vi "Process.vi"(8 "error in (no error)":errorcluster, 10 "pound in":refnum<class "Pound.lvclass">, 11 "qbus in":refnum<class "Qbus.lvclass">) -> (0 "error out":errorcluster)   [LabVIEW 2017, in "CmsAcquisition.lvlib"]
doc: "This process acquires waveforms from channels on NI 9230 and NI 9232 C Series modules. This process transfers data from a device-specific FPGA bitfile that reads samples directly from the FPGA at the sampling rate configured for the device."
uses:
  <vilib>/addons/InsightCM/Devices/Shared/Cms/CmsAcquisition/CmsAcquisition.lvlib
  <vilib>/addons/Qbus/Qbus.lvclass
  <vilib>/NI/Software Watchdog/Pound/Pound.lvclass
  <vilib>/addons/InsightCM/Devices/Shared/Cms/CmsAcquisition/controls/Configuration.ctl
  <vilib>/addons/InsightCM/Devices/Shared/Cms/CmsAcquisition/controls/TachometerConfig.ctl
  <vilib>/addons/InsightCM/Devices/Shared/Cms/CmsAcquisition/controls/FixedSizeArrays.ctl
  <vilib>/LabVIEW Targets/FPGA/cRIO/shared/nicrio_ModuleControls/nicrio_cRIO-9232_ConfigModeRing.ctl
  <vilib>/addons/InsightCM/Devices/Shared/Cms/cRIOWfmAcq/subVIs/RIO Wfm Cust Ctrls/rwfm_SamplingInfo.ctl
  <vilib>/addons/InsightCM/Devices/Shared/Cms/CmsAcquisition/controls/Group.ctl
  <vilib>/addons/InsightCM/Devices/Shared/Cms/CmsAcquisition/controls/Channel.ctl
  <vilib>/addons/InsightCM/Utilities/Analysis/Vibration/controls/HighPassFilterState.ctl
  <vilib>/addons/InsightCM/Devices/Shared/Cms/CmsAcquisition/controls/BurstMode.ctl
  <vilib>/addons/InsightCM/Devices/Shared/Cms/CmsAcquisition/controls/State.ctl
  <vilib>/addons/InsightCM/Devices/Shared/Common/DataFlow/controls/Type.ctl
  <vilib>/addons/InsightCM/Devices/Shared/Cms/CmsAcquisition/controls/StopAcquisitionResponse.ctl
  <vilib>/addons/InsightCM/Devices/Shared/Cms/cRIOWfmAcq/cRIOWfmLib.lvlib
  <vilib>/addons/TraceLogger/TraceLogger.lvlib
  <vilib>/NI/Software Watchdog/Watchdog/Watchdog.lvclass
  <vilib>/addons/InsightCM/Devices/Shared/Common/FpgaBitfileManager/FpgaBitfileManager.lvlib
  <vilib>/addons/InsightCM/Devices/Shared/Common/DataFlow/DataFlow.lvlib
  <vilib>/addons/InsightCM/Utilities/GlobalConfiguration/GlobalConfiguration.lvlib
  <vilib>/addons/InsightCM/Devices/Shared/Common/DataEventCreator/DataEventCreator.lvlib
  <vilib>/addons/InsightCM/Devices/Shared/Common/ServerComm/ServerComm.lvlib
  <vilib>/addons/InsightCM/Utilities/Analysis/Vibration/VibrationAnalysisFunctions.lvlib
  <vilib>/addons/InsightCM/Devices/Shared/Cms/CmsBurstMode/BurstMode.lvlib
  <vilib>/addons/InsightCM/Devices/Shared/Cms/CmsDataEventCreator/CmsDataEventCreator.lvlib
  <vilib>/addons/InsightCM/Devices/Shared/Cms/DAQmx/TSNcDAQ_AI.lvlib
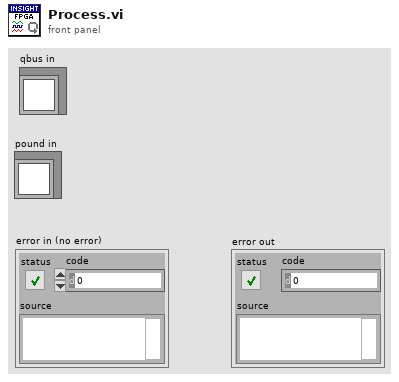
[diagram p1: front panel]
types:
  T1 = typedef "CmsAcquisition.lvlib/State.ctl" = enum16{"Unconfigured", "Configured", "Acquiring", "Stopped", "BurstMode"}
  T2 = typedef "CmsAcquisition.lvlib/Configuration.ctl" = cluster{"Acq":bool, "NumberOfModules":i16, "Dynamic FPGA VI Ref":refnum<k20>, "KeyphasorX3":T3[], "FixedSizeX32":T4, "SamplingInfo":T6, "Normal Mode Sample Rate":dbl, "BlockSize (sec)":dbl, "Samples To Read (per chan)":i32, "RunningAcquisitionLength":dbl, "Settling Time":dbl, "Fpga Tach Buffer Size (samples)":i32, "Waveform Groups":T7[], "Acquisition Block Number":i32, "Device Name":string, "ValidConfig":bool, "Last Dynamic Module":string, "HighPassFilterState":T9[], "Low Frequency Cutoff":dbl[], "BurstMode":T10, "DAQ task":refnum<k21>}
  T3 = typedef "CmsAcquisition.lvlib/TachometerConfig.ctl" = cluster{"slope":enum16{"falling", "rising"}, "threshold":dbl, "hysteresis":dbl}
  T4 = typedef "CmsAcquisition.lvlib/FixedSizeArrays.ctl" = cluster{"EnabledChannels":bool[], "Sensitivity":dbl[], "InputConfig":T5[]}
  T5 = typedef "nicrio_cRIO-9232_ConfigModeRing.ctl" = u8
  T6 = typedef "cRIOWfmLib.lvlib/rwfm_SamplingInfo.ctl" = cluster{"Number of Channels":i32, "Sampling Rate":dbl, "Channels":string[], "Units":string[], "Offsets":sgl[]}
  T7 = typedef "CmsAcquisition.lvlib/Group.ctl" = cluster{"Name":string, "Speed Reference":string, "Channels":T8[]}
  T8 = typedef "CmsAcquisition.lvlib/Channel.ctl" = cluster{"Name":string}
  T9 = typedef "VibrationAnalysisFunctions.lvlib/HighPassFilterState.ctl" = cluster{"designed":bool, "IIR Filter Cluster":cluster{"filter structure":enum32{"IIR 2nd Order", "IIR 4th Order"}, "Reverse Coefficients":dbl[], "Forward Coefficients":dbl[]}, "Filter State":dbl[]}
  T10 = typedef "CmsAcquisition.lvlib/BurstMode.ctl" = cluster{"Acquisition Time":dbl, "Sample Rate":dbl, "Collection Reason":string}
  T11 = typedef "DataFlow.lvlib/Type.ctl" = enum16{"High Rate", "Low Rate", "Burst Mode"}
  T12 = typedef "CmsAcquisition.lvlib/StopAcquisitionResponse.ctl" = cluster{"Reason":string, "Acquisition Stopped":bool, "State":variant}
  T13 = typedef "DataEventCreator.lvlib/RegisterDataSets.ctl" = cluster{"DataGroup":string, "DataSets":T14[]}
  T14 = typedef "CmsDataEventCreator.lvlib/DataSetRegistry.ctl" = cluster{"ChannelName":string, "DataSetType":T15, "DoNotWriteToDB":bool, "ParentName":string, "CalculateOnServer":bool}
  T15 = typedef "DataEvent.lvlib/DataSetType.ctl" = enum16{"Waveform", "SpeedProfile", "ThermalImage", "EmsaSweep"}
  T16 = typedef "DataFlow.lvlib/Data.ctl" = cluster{"DataGroup":string, "Waveforms":T17, "Map":T18, "Type":T11}
  T17 = typedef "wfmSGL_DVR.ctl" = refnum<data-value>
  T18 = typedef "PointValueMap.lvlib/PointMap.ctl" = refnum<data-value>
  T19 = typedef "CmsAcquisition.lvlib/StopAcquisitionRequest.ctl" = cluster{"Reason":string, "State":variant}
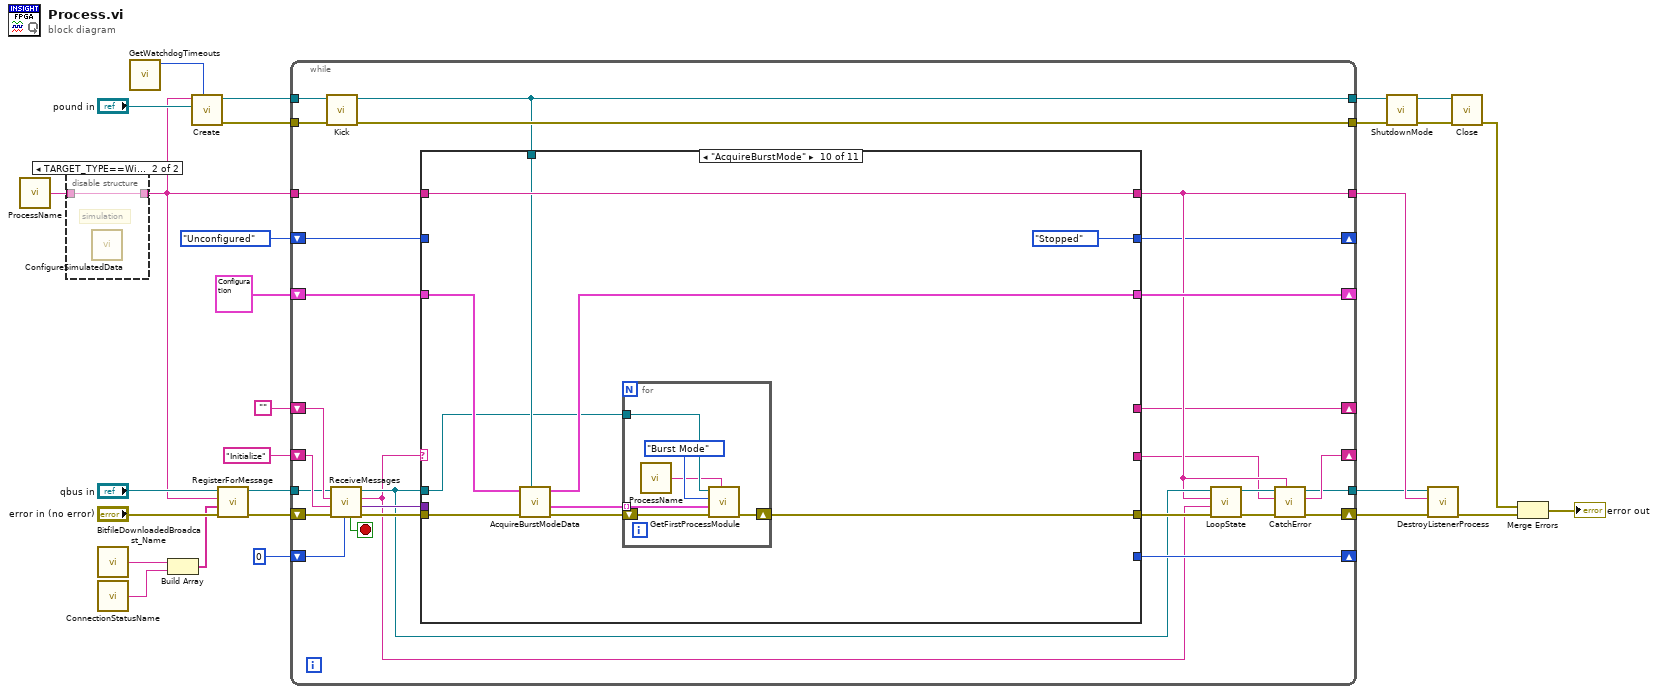
[diagram p0: block diagram]
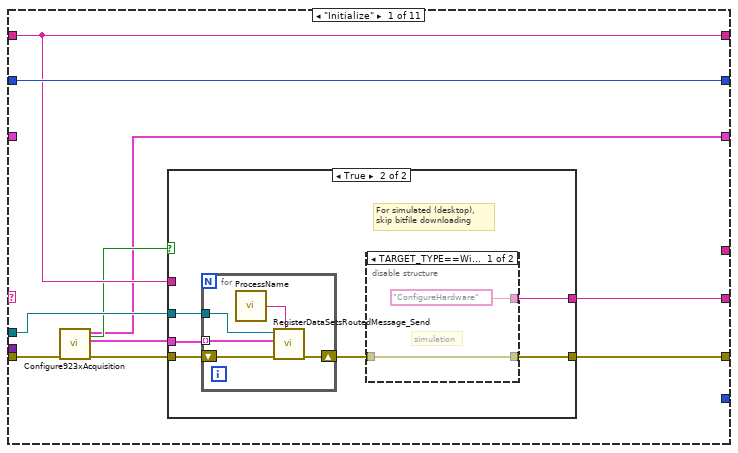
[diagram p3: hidden frame]
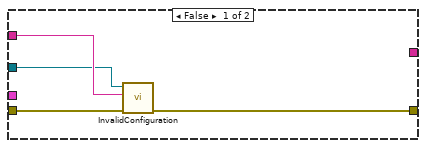
[diagram p4: hidden frame]
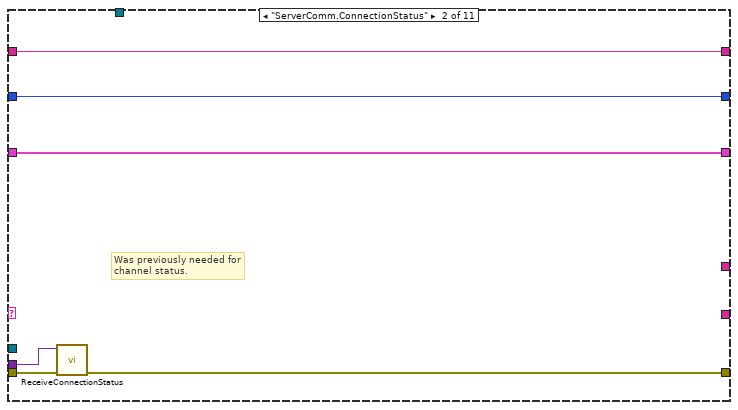
[diagram p6: hidden frame]
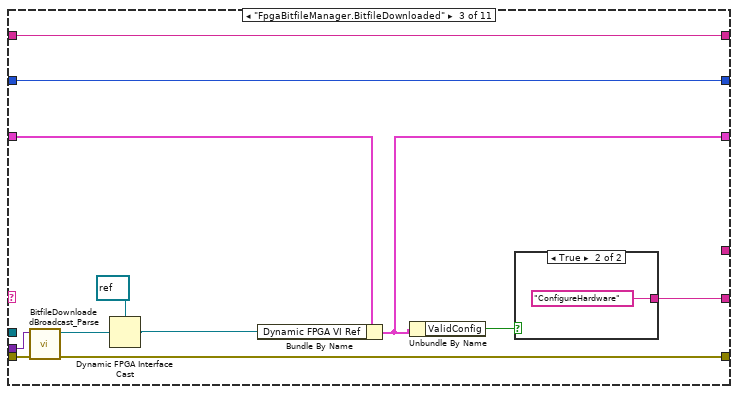
[diagram p7: hidden frame]
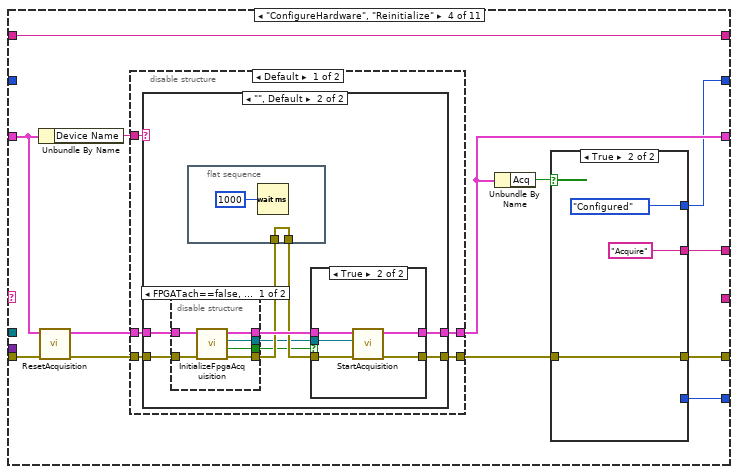
[diagram p9: hidden frame]
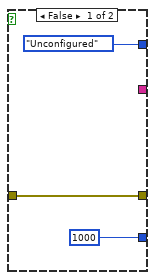
[diagram p10: hidden frame]
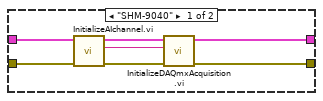
[diagram p11: hidden frame]
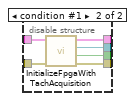
[diagram p13: hidden frame]
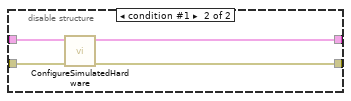
[diagram p14: hidden frame]
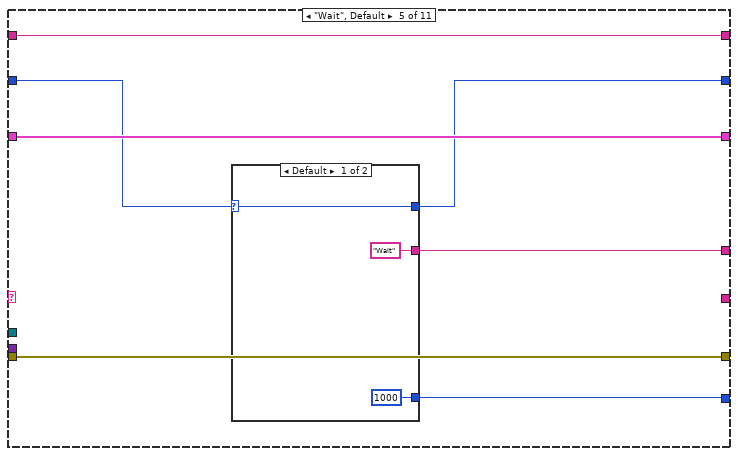
[diagram p15: hidden frame]
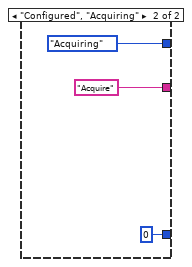
[diagram p16: hidden frame]
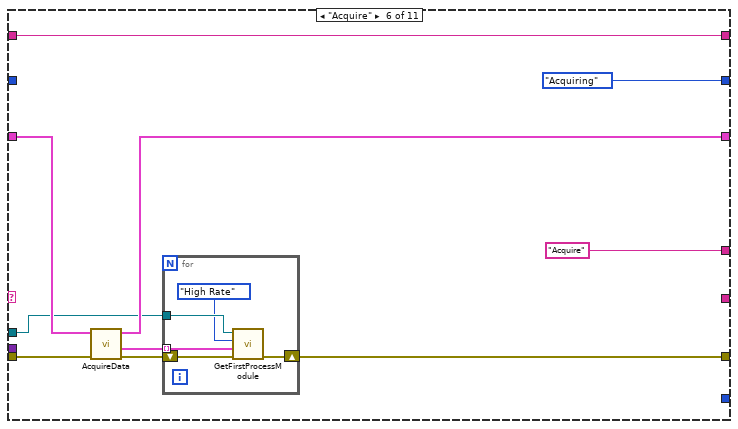
[diagram p17: hidden frame]
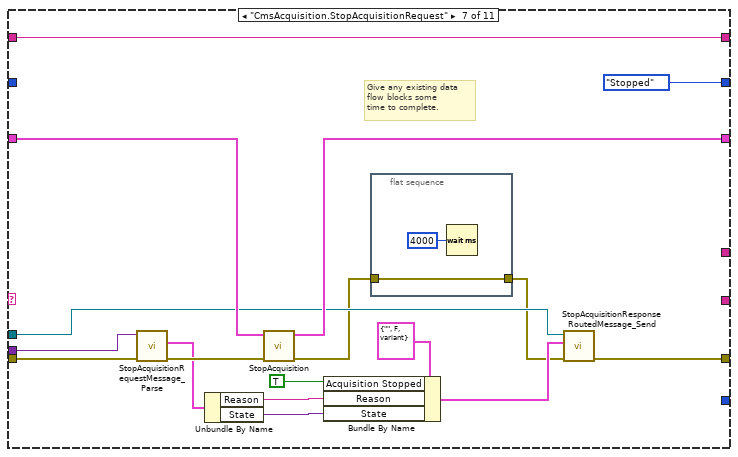
[diagram p18: hidden frame]
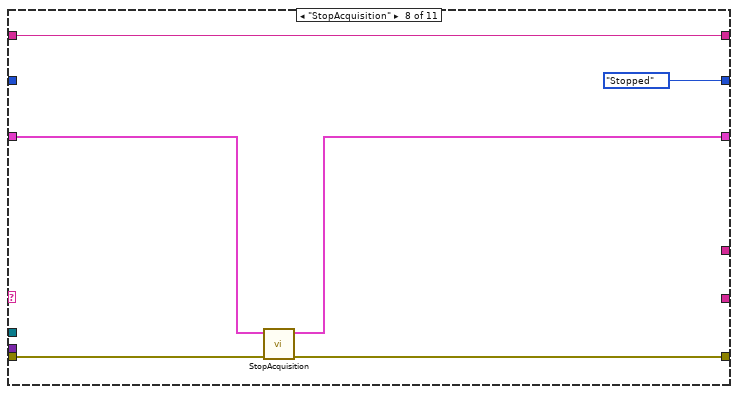
[diagram p19: hidden frame]
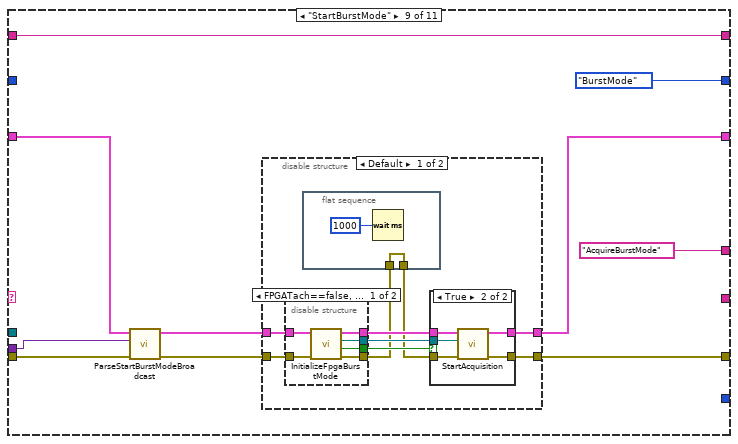
[diagram p20: hidden frame]
diagram:
  n1 = call <vilib>:"ProcessName.vi"() -> ("process name"=w6:string)  [unwired: 5 in]
  n2 = disable-structure shown="TARGET_TYPE==Windows" {
    disable-tunnel: [w29 w30] -> w7
    disable-tunnel: w6 -> [w29 w30]
    frame condition #0 (active) {
    }
    frame condition #1 {
      # "simulation"
      n3 = call <vilib>:"ConfigureSimulatedData.vi"() -> ()  [unwired: 12 in]
    }
  }
  n4 = call <vilib>:"BitfileDownloadedBroadcast_Name.vi"() -> ("message name"=w9:string)  [unwired: 5 in]
  n5 = call <vilib>:"ConnectionStatusName.vi"() -> ("message name"=w1:string)  [unwired: 5 in]
  n6 = call <vilib>:"GetWatchdogTimeouts.vi"() -> ("software timeout"=w2:u32)  [unwired: 10 in, 1 out]
  n7 = Build Array(w9, w1) -> (w10:string[])
  n8 = call <vilib>:"Create.vi"("Execution Timeout (ms)"=w2, "Pound"="pound in", "Name"=w7) -> ("error out"=w23:errorcluster, "Watchdog"=w24:refnum<data-value>)  [unwired: 7 in]
  n9 = call <vilib>:"RegisterForMessage.vi"("error in (no error)"="error in (no error)", "message names"=w10, "process name"=w7, "Qbus in"="qbus in") -> ("error in (no error)"=w12:errorcluster, "Qbus out"=w13:refnum<class "Qbus.lvclass">)  [unwired: 6 in]
  n10 = while {
    shift-right: [w46] -> w3
    shift-left: w12 -> [w53]
    shift-right: [w37] -> _
    shift-left: "" -> [w55]
    shift-right: [w59] -> _
    shift-left: T2 {"Acq"=FALSE, "NumberOfModules"=0, "Dynamic FPGA VI Ref"=refnum, "KeyphasorX3"=[], "FixedSizeX32"={"EnabledChannels"=[], "Sensitivity"=[], "InputConfig"=[]}, "SamplingInfo"={"Number of Channels"=4, "Sampling Rate"=4.0, "Channels"=[], "Units"=[], "Offsets"=[]}, "Normal Mode Sample Rate"=0.0, "BlockSize (sec)"=0.0, "Samples To Read (per chan)"=0, "RunningAcquisitionLength"=0.0, "Settling Time"=0.0, "Fpga Tach Buffer Size (samples)"=0, "Waveform Groups"=[], "Acquisition Block Number"=0, "Device Name"="", "ValidConfig"=FALSE, "Last Dynamic Module"="", "HighPassFilterState"=[], "Low Frequency Cutoff"=[], "BurstMode"={"Acquisition Time"=0.0, "Sample Rate"=0.0, "Collection Reason"=""}, "DAQ task"=""} ("Config out") -> [w58]
    shift-right: [w35] -> _
    shift-left: State."Unconfigured" ("loop state") -> [w57]
    shift-right: [w56] -> _
    shift-left: 0 ("milliseconds to wait") -> [w51]
    shift-right: [w44] -> _
    shift-left: "Initialize" -> [w54]
    tunnel: w13 -> [w52]
    tunnel: w7 -> [w32]
    tunnel: [w42] -> w4
    tunnel: [w38] -> w26
    tunnel: w24 -> [w41]
    tunnel: w23 -> [w40]
    tunnel: [w31] -> w20
    tunnel: [w39] -> w19
    stop <- w33 stop-if-true
    n11 = call <vilib>:"Kick.vi"("error in (no error)"=w40, "Watchdog"=w41) -> ("error out"=w39:errorcluster, "Watchdog"=w31:refnum<data-value>)  [unwired: 8 in]
    n12 = call <vilib>:"ReceiveMessages.vi"("timeout(100)"=w51, "error in (no error)"=w53, "priority action"=w54, "default action"=w55, "qbus in"=w52) -> ("error out"=w50:errorcluster, "msg value"=w49:variant, "action"=w34:string, "qbus out"=w45:refnum<class "Qbus.lvclass">, "exit"=w33:bool)  [unwired: 2 in]
    n13 = case shown="\"AcquireBurstMode\"" w34 {
      tunnel: w50 -> [w67 w91 w97 w110 w178 w188 w212 w219 w227 w275 w285]
      tunnel: [w63 w89 w96 w115 w178 w187 w203 w220 w232 w269 w286] -> w47
      tunnel: [_ _ _ w119 w176 "Acquire" _ _ "AcquireBurstMode" _ _] -> w37
      tunnel: [w60 w88 w95 w117 w177 w190 w214 w222 w231 w274 w287] -> w59
      tunnel: w58 -> [_ w88 w104 w108 w177 w191 w215 w223 w229 w276 w287]
      tunnel: w57 -> [w64 w92 w100 _ w173 _ _ _ _ _ _]
      tunnel: [_ _ _ w114 w174 _ _ _ _ _ _] -> w56
      tunnel: w32 -> [w62 w93 w105 w118 w175 w189 w216 w224 w234 w278 w288]
      tunnel: w49 -> [_ w90 w98 _ _ _ w213 _ w225 _ _]
      tunnel: w45 -> [w66 _ _ _ _ w186 w208 _ _ w270 _]
      tunnel: [w62 w93 w105 w118 w175 w189 w216 w224 w234 w278 w288] -> w38
      tunnel: [w65 _ w101 _ _ _ _ _ _ _ _] -> w36
      tunnel: [w64 w92 w100 w113 w172 State."Acquiring" ("loop state") State."Stopped" ("loop state") State."Stopped" ("loop state") State."BurstMode" ("loop state") State."Stopped" ("loop state") State."Unconfigured" ("loop state")] -> w35
      tunnel: w31 -> [_ _ _ _ _ _ _ _ _ w271 _]
      frame "Initialize" {
        n14 = call <vilib>:"Configure923xAcquisition.vi"("error in (no error)"=w67) -> ("error out"=w69:errorcluster, "register data sets"=w68:T13[], "923x Acquisition Config"=w60:T2, "valid"=w61:bool)  [unwired: 7 in]
        n15 = case shown="True" w61 {
          tunnel: w69 -> [w70 w79]
          tunnel: w68 -> [_ w78]
          tunnel: w66 -> [w71 w77]
          tunnel: [_ w76] -> w65
          tunnel: [w73 w75] -> w63
          tunnel: w62 -> [w72 _]
          frame False {
            n16 = call <vilib>:"InvalidConfiguration.vi"("error in (no error)"=w70, "description"=w72, "Qbus in"=w71) -> ("error out"=w73:errorcluster)  [unwired: 7 in, 1 out]
          }
          frame True {
            # "For simulated (desktop),\nskip bitfile downloading"
            n17 = for {
              shift-right: [w85] -> w74
              shift-left: w79 -> [w86]
              tunnel: w78 -> [w84] mode=indexing
              tunnel: w77 -> [w87]
              n18 = call <vilib>:"ProcessName.vi"() -> ("process name"=w83:string)  [unwired: 5 in]
              n19 = call <vilib>:"RegisterDataSetsRoutedMessage_Send.vi"("data event creator process name"=w83, "error in (no error)"=w86, "RegisterDataSet"=w84, "Qbus in"=w87) -> ("error out"=w85:errorcluster)  [unwired: 6 in, 1 out]
            }
            n20 = disable-structure shown="TARGET_TYPE==Windows" {
              disable-tunnel: w74 -> [w80 w82]
              disable-tunnel: [w80 w82] -> w75
              disable-tunnel: ["ConfigureHardware" _] -> w76
              frame condition #0 {
                # "simulation"
              }
              frame condition #1 (active) {
              }
            }
          }
        }
      }
      frame "ServerComm.ConnectionStatus" {
        # "Was previously needed for\nchannel status."
        n21 = call <vilib>:"ReceiveConnectionStatus.vi"("error in (no error)"=w91, "body"=w90) -> ("error out"=w89:errorcluster)  [unwired: 6 in, 3 out]
      }
      frame "FpgaBitfileManager.BitfileDownloaded" {
        n22 = call <vilib>:"BitfileDownloadedBroadcast_Parse.vi"("error in (no error)"=w97, "data"=w98) -> ("error out"=w96:errorcluster, "FPGA reference"=w99:refnum<k20>)  [unwired: 8 in]
        n23 = Dynamic FPGA Interface Cast(Session In=refnum<k20> refnum ("Dynamic FPGA VI Ref"), Type=w99) -> (Session Out=w103:refnum<k20>)
        n24 = Bundle By Name(cluster=w104, "Dynamic FPGA VI Ref"=w103) -> (w95:T2)
        n25 = Unbundle By Name(w95) -> ("ValidConfig"=w94:bool)
        n26 = case shown="True" w94 {
          tunnel: [_ "ConfigureHardware"] -> w101
          frame False {
          }
          frame True {
          }
        }
      }
      frame "ConfigureHardware", "Reinitialize" {
        n27 = Unbundle By Name(w108) -> ("Device Name"=w107:string)
        n28 = call <vilib>:"ResetAcquisition.vi"("error in (no error)"=w110, "config in"=w108) -> ("error out"=w109:errorcluster, "config out"=w111:T2)  [unwired: 8 in]
        n29 = disable-structure shown="Default" {
          disable-tunnel: w111 -> [w128 w169]
          disable-tunnel: w109 -> [w130 w171]
          disable-tunnel: [w129 w170] -> w116
          disable-tunnel: [w127 w168] -> w117
          disable-tunnel: w107 -> [w126 _]
          frame condition #0 (active) {
            n30 = case shown="\"\", Default" w126 {
              tunnel: w130 -> [w137 w146]
              tunnel: [w132 w145] -> w129
              tunnel: w128 -> [w136 w139]
              tunnel: [w131 w138] -> w127
              frame "SHM-9040" {
                n31 = call <vilib>:"InitializeAIchannel.vi.vi"("error in (no error)"=w137, "config in"=w136) -> ("error out"=w133:errorcluster, "cDAQ with TSN AI Channel(s)"=w134:tag, "config out"=w135:T2)  [unwired: 7 in]
                n32 = call <vilib>:"InitializeDAQmxAcquisition.vi.vi"("error in"=w133, "cDAQ with TSN AI Channel(s)"=w134, "config in"=w135) -> ("error out"=w132:errorcluster, "config out"=w131:T2)  [unwired: 7 in]
              }
              frame "", Default {
                n33 = disable-structure shown="FPGATach==false, Default" {
                  disable-tunnel: w146 -> [w161 w167]
                  disable-tunnel: [w160 w165] -> w143
                  disable-tunnel: w139 -> [w159 w166]
                  disable-tunnel: [w158 w164] -> w144
                  disable-tunnel: [w157 w163] -> w141
                  disable-tunnel: [w156 w162] -> w140
                  frame condition #0 (active) {
                    n34 = call <vilib>:"InitializeFpgaAcquisition.vi"("error in (no error)"=w161, "923x Acquisition Config"=w159) -> ("error out"=w160:errorcluster, "start acquisition?"=w156:bool, "dynamic FPGA VI reference"=w157:refnum<k20>, "923x Acquisition Config out"=w158:T2)  [unwired: 6 in]
                  }
                  frame condition #1 {
                    n35 = call <vilib>:"InitializeFpgaWithTachAcquisition.vi"("error in (no error)"=w167, "923x Acquisition Config"=w166) -> ("error out"=w165:errorcluster, "start acquisition?"=w162:bool, "dynamic FPGA VI reference"=w163:refnum<k20>, "923x Acquisition Config out"=w164:T2)  [unwired: 6 in]
                  }
                }
                n36 = flat-sequence {
                  tunnel: [w147] -> w142
                  tunnel: w143 -> [w147]
                  frame #0 {
                    n37 = Wait (ms)(milliseconds to wait=u32 1000) -> ()  [unwired: 1 out]
                  }
                }
                n38 = case shown="True" w140 {
                  tunnel: [w150 w155] -> w145
                  tunnel: w142 -> [w150 w154]
                  tunnel: w144 -> [w149 w152]
                  tunnel: w141 -> [_ w151]
                  tunnel: [w149 w153] -> w138
                  frame False {
                  }
                  frame True {
                    n39 = call <vilib>:"StartAcquisition.vi"("error in (no error)"=w154, "fpga ref"=w151, "923x Acquisition Config in"=w152) -> ("error out"=w155:errorcluster, "923x Acquisition Config out"=w153:T2)  [unwired: 7 in]
                  }
                }
              }
            }
          }
          frame condition #1 {
            n40 = call <vilib>:"ConfigureSimulatedHardware.vi"("error in (no error)"=w171, "configuration"=w169) -> ("error out"=w170:errorcluster, "configuration out"=w168:T2)  [unwired: 8 in]
          }
        }
        n41 = Unbundle By Name(w117) -> ("Acq"=w112:bool)
        n42 = case shown="True" w112 {
          tunnel: [_ "Acquire"] -> w119
          tunnel: [w122 w124] -> w115
          tunnel: w116 -> [w122 w124]
          tunnel: [1000 _] -> w114
          tunnel: [State."Unconfigured" ("loop state") State."Configured" ("loop state")] -> w113
          frame False {
          }
          frame True {
          }
        }
      }
      frame "Wait", Default {
        n43 = case shown="Default" w173 {
          selector: w173 -> [w179 _]
          tunnel: ["Wait" "Acquire"] -> w176
          tunnel: [1000 0] -> w174
          tunnel: [w179 State."Acquiring" ("loop state")] -> w172
          frame Default {
          }
          frame "Configured", "Acquiring" {
          }
        }
      }
      frame "Acquire" {
        n44 = call <vilib>:"AcquireData.vi"("error in (no error)"=w188, "923x acquisition config"=w191) -> ("error out"=w193:errorcluster, "dataflow messages"=w192:T16[], "923x acquisition config out"=w190:T2)  [unwired: 7 in]
        n45 = for {
          tunnel: w192 -> [w196] mode=indexing
          tunnel: w186 -> [w197]
          shift-right: [w198] -> w187
          shift-left: w193 -> [w199]
          n46 = call <vilib>:"GetFirstProcessModule.vi"("error in (no error)"=w199, "data"=w196, "type"=Type."High Rate", "Qbus in"=w197) -> ("error out"=w198:errorcluster)  [unwired: 6 in, 1 out]
        }
      }
      frame "CmsAcquisition.StopAcquisitionRequest" {
        # "Give any existing data\nflow blocks some\ntime to complete."
        n47 = call <vilib>:"StopAcquisitionRequestMessage_Parse.vi"("error in (no error)"=w212, "message"=w213) -> ("error out"=w211:errorcluster, "StopAcquisitionRequest"=w210:T19)  [unwired: 8 in]
        n48 = Unbundle By Name(w210) -> ("Reason"=w205:string, "State"=w200:variant)
        n49 = call <vilib>:"StopAcquisition.vi"("error in (no error)"=w211, "config"=w215) -> ("error out"=w201:errorcluster, "config out"=w214:T2)  [unwired: 8 in]
        n50 = Bundle By Name(cluster=T12 {"Reason"="", "Acquisition Stopped"=FALSE, "State"=variant} ("Stop Acquisition Response"), "Acquisition Stopped"=TRUE, "Reason"=w205, "State"=w200) -> (w207:T12)
        n51 = flat-sequence {
          tunnel: [w218] -> w202
          tunnel: w201 -> [w218]
          frame #0 {
            n52 = Wait (ms)(milliseconds to wait=u32 4000) -> ()  [unwired: 1 out]
          }
        }
        n53 = call <vilib>:"StopAcquisitionResponseRoutedMessage_Send.vi"("error in (no error)"=w202, "Stop Acquisition Response"=w207, "Qbus in"=w208) -> ("error out"=w203:errorcluster)  [unwired: 7 in, 1 out]
      }
      frame "StopAcquisition" {
        n54 = call <vilib>:"StopAcquisition.vi"("error in (no error)"=w219, "config"=w223) -> ("error out"=w220:errorcluster, "config out"=w222:T2)  [unwired: 8 in]
      }
      frame "StartBurstMode" {
        n55 = call <vilib>:"ParseStartBurstModeBroadcast.vi"("error in (no error)"=w227, "msg value"=w225, "config"=w229) -> ("error out"=w226:errorcluster, "config out"=w228:T2)  [unwired: 7 in]
        n56 = disable-structure shown="Default" {
          disable-tunnel: w226 -> [w243 w265]
          disable-tunnel: w228 -> [w242 w266]
          disable-tunnel: [w239 w267] -> w232
          disable-tunnel: [w238 w268] -> w231
          frame condition #0 (active) {
            n57 = disable-structure shown="FPGATach==false, Default" {
              disable-tunnel: w243 -> [w257 w262]
              disable-tunnel: [w256 w261] -> w236
              disable-tunnel: w242 -> [w258 w263]
              disable-tunnel: [w253 w264] -> w240
              disable-tunnel: [w254 w259] -> w241
              disable-tunnel: [w255 w260] -> w237
              frame condition #0 (active) {
                n58 = call <vilib>:"InitializeFpgaBurstMode.vi"("error in (no error)"=w257, "923x Acquisition Config"=w258) -> ("error out"=w256:errorcluster, "start acquisition?"=w255:bool, "dynamic FPGA VI reference"=w254:refnum<k20>, "923x Acquisition Config out"=w253:T2)  [unwired: 6 in]
              }
              frame condition #1 {
                n59 = call <vilib>:"InitializeFpgaWithTachBurstMode.vi"("error in (no error)"=w262, "923x Acquisition Config"=w263) -> ("error out"=w261:errorcluster, "start acquisition?"=w260:bool, "dynamic FPGA VI reference"=w259:refnum<k20>, "923x Acquisition Config out"=w264:T2)  [unwired: 6 in]
              }
            }
            n60 = flat-sequence {
              tunnel: [w244] -> w235
              tunnel: w236 -> [w244]
              frame #0 {
                n61 = Wait (ms)(milliseconds to wait=u32 1000) -> ()  [unwired: 1 out]
              }
            }
            n62 = case shown="True" w237 {
              tunnel: w235 -> [w246 w252]
              tunnel: w241 -> [_ w251]
              tunnel: w240 -> [w247 w250]
              tunnel: [w246 w249] -> w239
              tunnel: [w247 w248] -> w238
              frame False {
              }
              frame True {
                n63 = call <vilib>:"StartAcquisition.vi"("error in (no error)"=w252, "fpga ref"=w251, "923x Acquisition Config in"=w250) -> ("error out"=w249:errorcluster, "923x Acquisition Config out"=w248:T2)  [unwired: 7 in]
              }
            }
          }
          frame condition #1 {
            n64 = call <vilib>:"ConfigureSimulatedBurstMode.vi"("error in (no error)"=w265, "config in"=w266) -> ("error out"=w267:errorcluster, "configuration out"=w268:T2)  [unwired: 8 in]
          }
        }
      }
      frame "AcquireBurstMode" {
        n65 = call <vilib>:"AcquireBurstModeData.vi"("Watchdog"=w271, "error in (no error)"=w275, "config in"=w276) -> ("error out"=w273:errorcluster, "burst mode dataflow messages"=w277:T16[], "config out"=w274:T2)  [unwired: 6 in]
        n66 = for {
          tunnel: w277 -> [w281] mode=indexing
          tunnel: w270 -> [w282]
          shift-right: [w283] -> w269
          shift-left: w273 -> [w284]
          n67 = call <vilib>:"ProcessName.vi"() -> ("process name"=w279:string)  [unwired: 5 in]
          n68 = call <vilib>:"GetFirstProcessModule.vi"("originator"=w279, "error in (no error)"=w284, "data"=w281, "type"=Type."Burst Mode", "Qbus in"=w282) -> ("error out"=w283:errorcluster)  [unwired: 5 in, 1 out]
        }
      }
      frame "Exit" {
        n69 = call <vilib>:"StopAcquisition.vi"("error in (no error)"=w285, "config"=w287) -> ("error out"=w286:errorcluster)  [unwired: 8 in, 1 out]
      }
    }
    n70 = call <vilib>:"LoopState.vi"("error in (no error)"=w47, "loop action"=w34, "process name"=w38, "Qbus in"=w45) -> ("error out"=w48:errorcluster, "Qbus out"=w43:refnum<class "Qbus.lvclass">)  [unwired: 6 in]
    n71 = call <vilib>:"CatchError.vi"("source"=w38, "error in (no error)"=w48, "next action in"=w36, "Qbus in"=w43) -> ("error out"=w46:errorcluster, "next action out"=w44:string, "Qbus out"=w42:refnum<class "Qbus.lvclass">)  [unwired: 5 in]
  }
  n72 = call <vilib>:"ShutdownMode.vi"("error in (no error)"=w19, "Watchdog"=w20) -> ("error out"=w21:errorcluster, "Watchdog"=w22:refnum<data-value>)  [unwired: 8 in]
  n73 = call <vilib>:"DestroyListenerProcess.vi"("error in (no error)"=w3, "process name"=w26, "Qbus in"=w4) -> ("error in (no error)"=w17:errorcluster)  [unwired: 7 in, 1 out]
  n74 = call <vilib>:"Close.vi"("error in (no error)"=w21, "Watchdog"=w22) -> ("error out"=w16:errorcluster)  [unwired: 9 in]
  n75 = Merge Errors(w16, w17) -> (→"error out":errorcluster)
